vi "AddToMissionArray.vi"() -> ()   [LabVIEW 2013]
uses:
  Data/TypeDefs/UTM Location.ctl
  Data/TypeDefs/MissionTypeControl.ctl
  Classes/Missions/GenericMission/GenericMission.lvclass
  Classes/Missions/GoTo/GoTo.lvclass
  Classes/Missions/RoundBouy/RoundBouy.lvclass
  Classes/Missions/PassBouy/PassBouy.lvclass
  Classes/Missions/StationKeeping/StationKeeping.lvclass
panel:
  in  "DeleteMission":bool
  in  "Mission Type":T1
  in  "Points of Interest":T2[](array[typedef]) {"North" format="%#_10f"; "East" format="%#_8f"}
  in  "Tolerance (m)":dbl
  in  "Duration (s)":dbl=-1.0
  in  "Timeout (s)":dbl=-1.0
  in  "CreateMission":bool
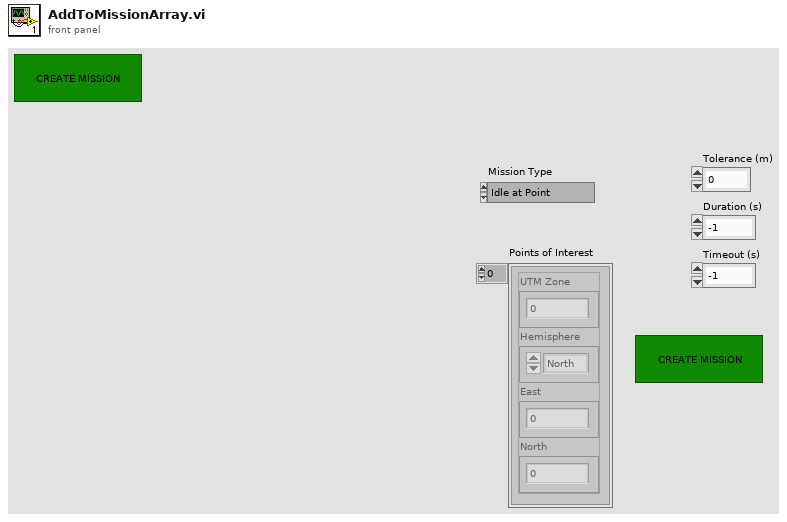
[diagram p1: front panel]
types:
  T1 = typedef "MissionTypeControl.ctl" = enum16{"Idle at Point", "Drive to Waypoint", "Round Buoy to Port", "Round Buoy to Starboard", "Pass Between Buoys", "Station Keeping"}
  T2 = typedef "UTM Location.ctl" = cluster{"UTM Zone":dbl, "Hemisphere":enum16{"North", "South"}, "East":dbl, "North":dbl}
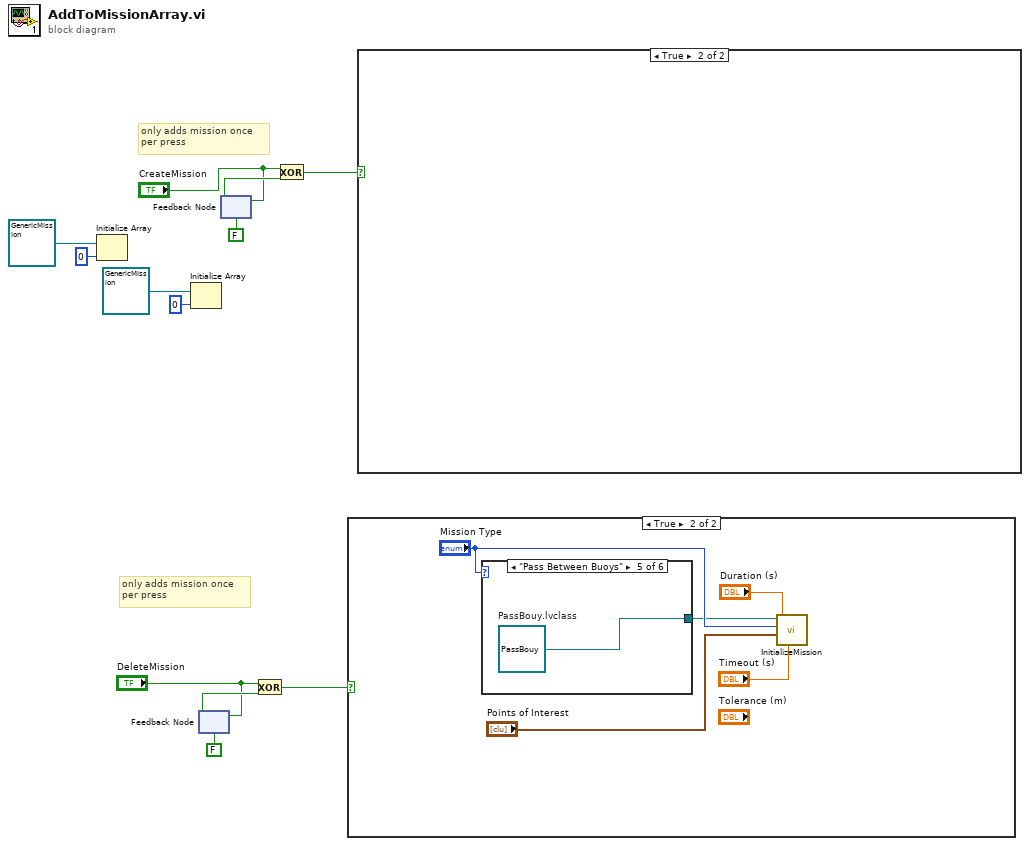
[diagram p0: block diagram]
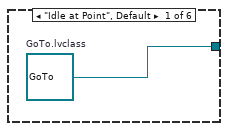
[diagram p3: hidden frame]
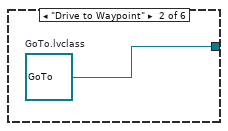
[diagram p4: hidden frame]
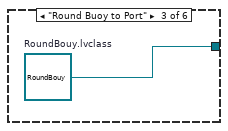
[diagram p5: hidden frame]
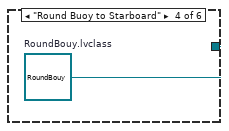
[diagram p6: hidden frame]
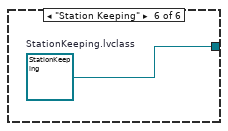
[diagram p7: hidden frame]
diagram:
  # "only adds mission once \nper press"
  # "only adds mission once \nper press"
  n1 = Initialize Array(refnum<class "GenericMission.lvclass"> refnum ("GenericMission.lvclass"), 0 ("dimension size")) -> ()  [unwired: 1 out]
  n2 = Initialize Array(refnum<class "GenericMission.lvclass"> refnum ("GenericMission.lvclass"), 0 ("dimension size")) -> ()  [unwired: 1 out]
  n3 = feedback #1(FALSE) -> (w5:bool)
  n4 = feedback-in #1("DeleteMission") -> ()
  n5 = feedback #2(FALSE) -> (w9:bool)
  n6 = feedback-in #2("CreateMission") -> ()
  n7 = Exclusive Or(1:w5, 2:"DeleteMission") -> (0:w3:bool)
  n8 = Exclusive Or(1:w9, 2:"CreateMission") -> (0:w8:bool)
  n9 = case shown="True" w3 {
    frame False {
    }
    frame True {
      n10 = case shown="\"Pass Between Buoys\"" "Mission Type" {
        tunnel: [w18 w19 w20 w21 w22 w23] -> w13
        frame "Idle at Point", Default {
          w18 = refnum<class "GoTo.lvclass"> refnum  # GoTo.lvclass
        }
        frame "Drive to Waypoint" {
          w19 = refnum<class "GoTo.lvclass"> refnum  # GoTo.lvclass
        }
        frame "Round Buoy to Port" {
          w20 = refnum<class "RoundBouy.lvclass"> refnum  # RoundBouy.lvclass
        }
        frame "Round Buoy to Starboard" {
          w21 = refnum<class "RoundBouy.lvclass"> refnum  # RoundBouy.lvclass
        }
        frame "Pass Between Buoys" {
          w22 = refnum<class "PassBouy.lvclass"> refnum  # PassBouy.lvclass
        }
        frame "Station Keeping" {
          w23 = refnum<class "StationKeeping.lvclass"> refnum  # StationKeeping.lvclass
        }
      }
      n11 = call-dynamic "InitializeMission.vi"("Timeout (s)"="Timeout (s)", "Duration (s)"="Duration (s)", "Points of Interest"="Points of Interest", "Mission Type"="Mission Type", "GenericMission in"=w13) -> ()  [unwired: 5 in, 2 out]
    }
  }
  n12 = case shown="True" w8 {
    frame False {
    }
    frame True {
    }
  }
